vi "configuration UI.vi"() -> ()   [LabVIEW 2015, in "TDMS datalogger editor node.lvclass"]
uses:
  TDMS datalogger editor node.lvclass
  <vilib>/NI/Configuration Framework/Node/NodeRef.ctl
  <vilib>/NI/Configuration Framework/Node/NISE_CEF_Node.lvclass
  <vilib>/NI/AMC/Message Queue.ctl
  <vilib>/NI/AMC/Message.ctl
  <vilib>/NI/Tools/Keyed Array/KeyedArray.ctl
  <vilib>/NI/Configuration Framework/Node/UserEventRef.ctl
  <vilib>/NI/Configuration Framework/Controls/EventCluster.ctl
  <vilib>/NI/DCAF UI Toolkit/Controls/Move One Right.ctl
  <vilib>/NI/DCAF UI Toolkit/Controls/Move All Right.ctl
  <vilib>/NI/DCAF UI Toolkit/Controls/Move One Left.ctl
  <vilib>/NI/Configuration Framework/Node/NodeChangeEvent.ctl
  <vilib>/NI/DCAF UI Toolkit/Controls/Add.ctl
  <vilib>/NI/DCAF UI Toolkit/Controls/Remove.ctl
  <vilib>/NI/Configuration Framework/Node/RefreshUIEvent.ctl
  <vilib>/NI/Configuration Framework/Node/StopEvent.ctl
  <vilib>/NI/Configuration Framework/Node/CacheState.ctl
  <vilib>/NI/DCAF/Tag Editor Core/Table API/Available Tag Menu/channel action event.ctl
  <vilib>/NI/DCAF/Tag Editor Core/Table API/Available Tag Menu/dialog output action.ctl
  <vilib>/NI/Tag Bus Module Framework/channel/TBM channel.lvclass
  <vilib>/NI/Tag Bus/tag/tag descriptor.lvclass
  <vilib>/NI/DCAF/Tag Editor Core/Table API/Table Manager/Call Back Ref Type Def.ctl
  <vilib>/NI/DCAF/Tag Editor Core/Configuration Editor/Classes/Engine Parent/Engine Parent Editor Node.lvclass
  <vilib>/NI/DCAF/Tag Editor Core/Configuration Editor/Classes/Module editor node/module editor node.lvclass
  <vilib>/NI/DCAF UI Toolkit/Controls/Configure.ctl
  <vilib>/NI/DCAF/Tag Editor Core/Table API/Table Manager/object ref.ctl
  module/configuration/TDMS datalogger configuration.lvclass
  <vilib>/NI/DCAF/Tag Editor Core/Table API/Table Manager/references.ctl
  <vilib>/Utility/miscctls.llb/LVPositionTypeDef.ctl
  TDMS datalogger editor node.lvclass/TDMS datalogger editor node.ctl
  module/configuration/TDMS datalogger configuration.lvclass/TDMS datalogger configuration.ctl
  Write channel table.vi
  Write avail tags table.vi
  module/configuration/Read backup directory.vi
  module/configuration/Read Path.vi
  module/configuration/Read queue size.vi
  module/configuration/Read scans per write.vi
  module/configuration/Read add enable channel.vi
  module/configuration/Read channel pattern matches.vi
  module/configuration/Read log name.vi
  module/configuration/Read logrotate_options.vi
  <vilib>/NI/DCAF/Tag Editor Core/Configuration Editor/Classes/Module editor node/Read Module Configuration.vi
  <vilib>/NI/Tag Bus Module Framework/module configuration/TBM module configuration.lvclass
  <vilib>/NI/DCAF/Tag Editor Core/Table API/Listbox/Multi Column Listbox.lvclass
  <vilib>/NI/Configuration Framework/NISE_CEF_TreeControl.lvlib
  <vilib>/NI/DCAF UI Toolkit/Controls/DCAF UI Elements.lvlib
  <vilib>/NI/Tools/Keyed Array/Tools_KeyedArray.lvlib
  <vilib>/NI/AMC/AMC.lvlib
  <vilib>/NI/DCAF/Tag Editor Core/Table API/Table Manager/Table Manager.lvclass
  <vilib>/NI/DCAF/Tag Editor Core/Table API/Table Manager.lvlib
panel:
  in  "References":T1
  in  "Maximum File Size (KB)":i64=10000
  in  "user event out":refnum<user-event>
  in  "cache state":T2
  in  "stop event":T3
  in  "refresh UI":T4
  in  "node change":T5
  in  "Tab Control":T6(tab)
  in  "channels":i32(listbox)
  in  "remove":T7
  in  "avail tags":i32(listbox)=-1
  in  "add all":T8
  in  "add1":T9
  out "Logging File Path":string
  in  "file name error":bool
  in  "Log Directory":string
  in  "File Name":string
  out "Enable Tag":string
  in  "path error":bool
  in  "Use Enable Channel":bool
  in  "recalc":bool
  out "Approximate Memory Usage":dbl
  in  "Queue Size":u16=2
  in  "Scans Per Write":u16=20
  in  "Log Directory":path
  in  "Maximum Age of Files (days)":dbl=365.0
  in  "Rotate count":u32 caption="Maximum Number of Archived Files To Keep"
  in  "archive in place":bool caption="Archive Old Logs in Original Directory"
  in  "Archive Directory":string
  in  "Archive Directory":path
  in  "archive error":bool
  in  "Channel Subscription Pattern Matches":string[](array[string])
  in  "Enable Dynamic Mapping":bool
  in  "Remove Group":T10
  in  "Add Group":T11
  in  "Remove from Group":T9
  in  "Add to Group":T7
  in  "avail logged tags":i32(listbox)=-1
  in  "Groups":string(tree)="Channel1"
  in  "Add Group Name":string caption="File Name"
  in  "File Property Settings":T12
  in  "File Properties":i32(listbox)
  in  "Add File Property":T11
  in  "Remove File Property":T10
  in  "user event":T13
  in  "main queue":T14
  in  "node ref":T15
  # "kB"
  # "Note: This value ignores dynamic mapping"
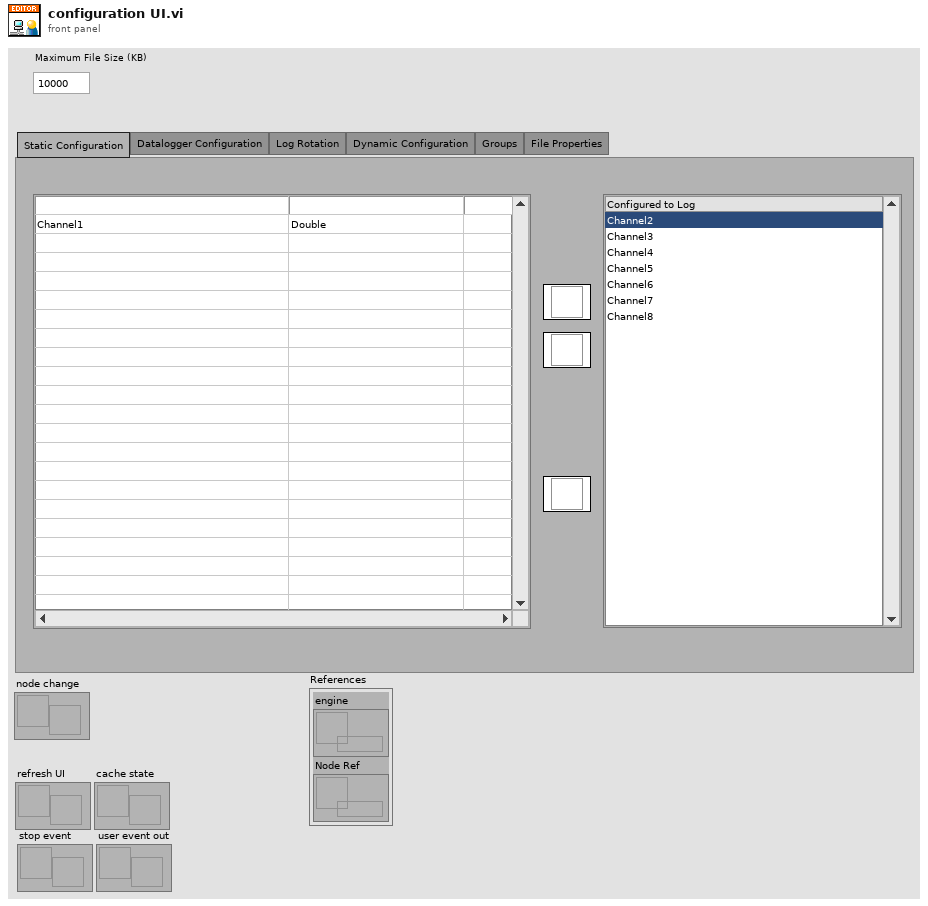
[diagram p1: front panel]
types:
  T1 = typedef "Table Manager.lvlib/Table Manager.lvclass/object ref.ctl" = cluster{"engine":refnum<data-value>, "Node Ref":refnum<data-value>}
  T2 = typedef "NISE_CEF_Node.lvclass/CacheState.ctl" = refnum<user-event>
  T3 = typedef "NISE_CEF_Node.lvclass/StopEvent.ctl" = refnum<user-event>
  T4 = typedef "NISE_CEF_Node.lvclass/RefreshUIEvent.ctl" = refnum<user-event>
  T5 = typedef "NISE_CEF_Node.lvclass/NodeChangeEvent.ctl" = refnum<user-event>
  T6 = enum32{"Static Configuration", "Datalogger Configuration", "Log Rotation", "Dynamic Configuration", "Groups", "File Properties"}
  T7 = typedef "DCAF UI Elements.lvlib/Move One Left.ctl" = bool
  T8 = typedef "DCAF UI Elements.lvlib/Move All Right.ctl" = bool
  T9 = typedef "DCAF UI Elements.lvlib/Move One Right.ctl" = bool
  T10 = typedef "DCAF UI Elements.lvlib/Remove.ctl" = bool
  T11 = typedef "DCAF UI Elements.lvlib/Add.ctl" = bool
  T12 = typedef "DCAF UI Elements.lvlib/Configure.ctl" = bool
  T13 = typedef "NISE_CEF_Node.lvclass/UserEventRef.ctl" = refnum<user-event>
  T14 = typedef "AMC.lvlib/Message Queue.ctl" = refnum<queue>
  T15 = typedef "NISE_CEF_Node.lvclass/NodeRef.ctl" = refnum<data-value>
  T16 = typedef "Table Manager.lvlib/Table Manager.lvclass/references.ctl" = cluster{"stop event":T3, "refresh UI":T4, "cache state":T2, "node change":T5, "user event out":refnum<user-event>, "main queue":T14, "user event":T13}
  T17 = typedef "LVPositionTypeDef.ctl" = cluster{"Left":i32, "Top":i32}
  T18 = typedef "TBM configuration.lvclass/Target Types.ctl" = enum16{"Windows", "Mac", "Linux", "Linux RT ARM", "VxWorks", "Pharlap", "Other", "Linux RT x64"}
  T19 = typedef "LogRotate.lvclass/options.ctl" = cluster{"max file size (bytes)":i64, "rotate count":u32, "max age (days)":dbl, "No archive dir":bool, "Archive dir":path}
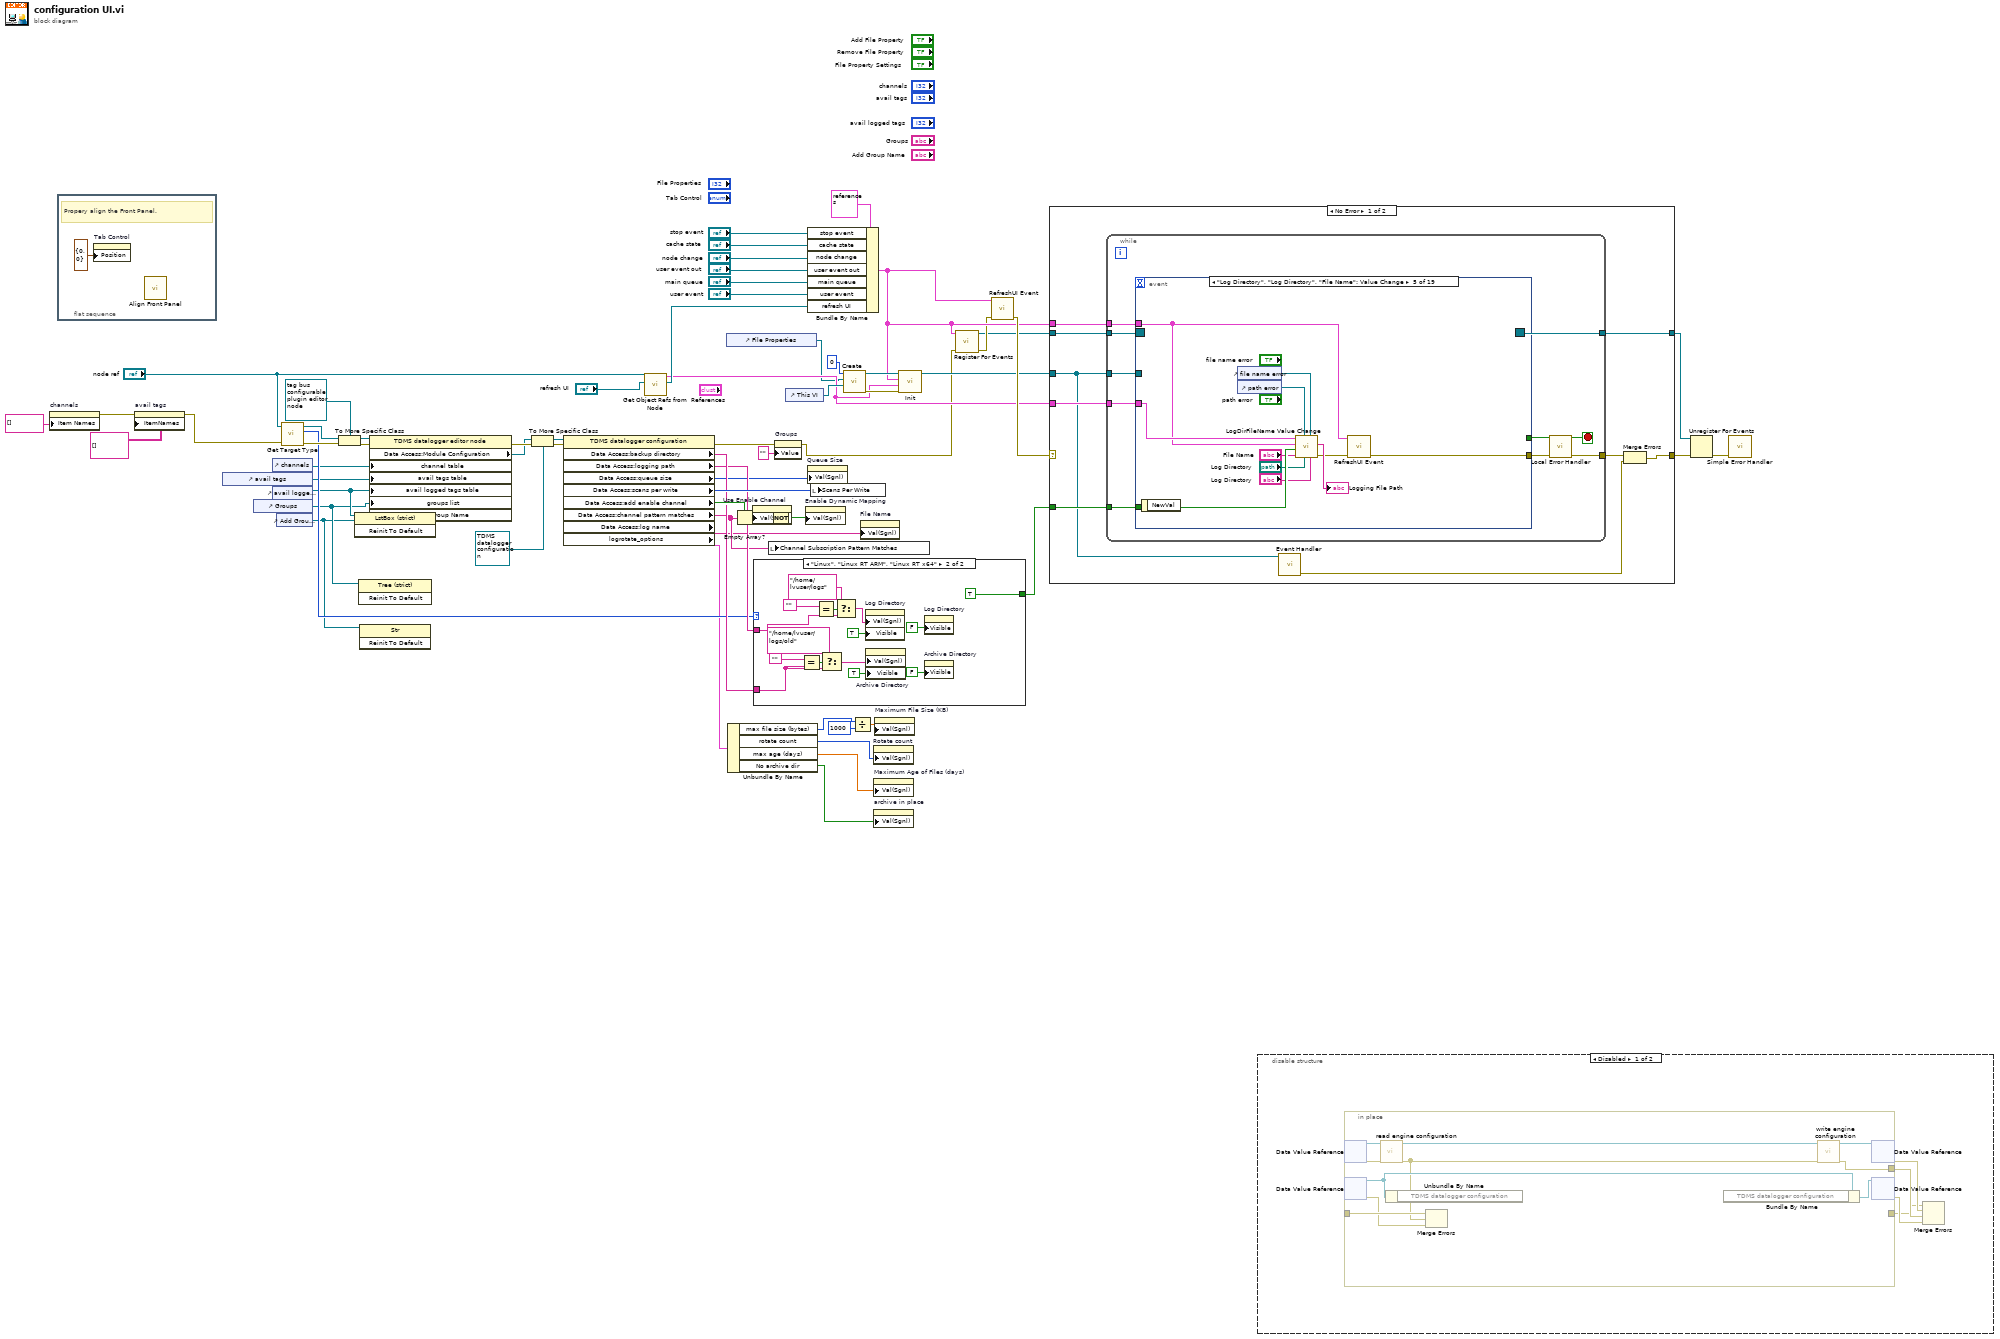
[diagram p0: block diagram]
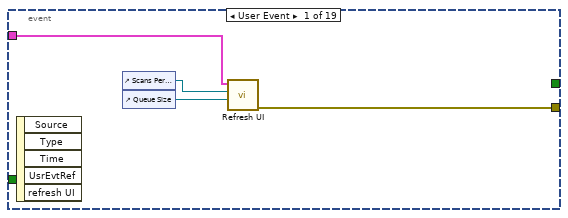
[diagram p2: hidden frame]
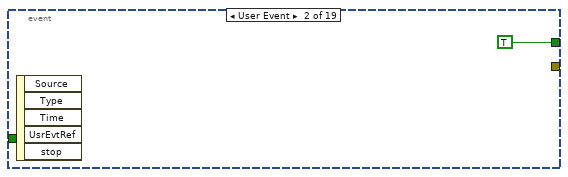
[diagram p3: hidden frame]
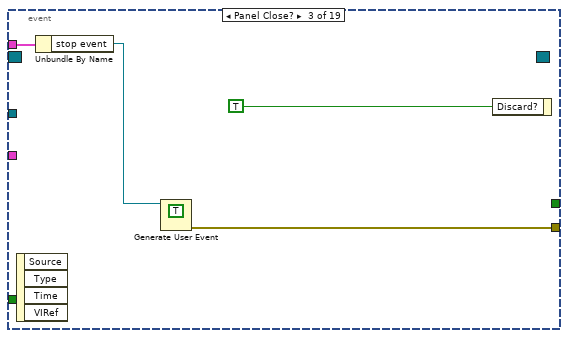
[diagram p4: hidden frame]
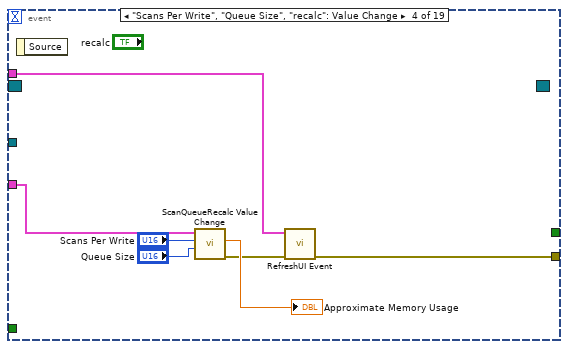
[diagram p5: hidden frame]
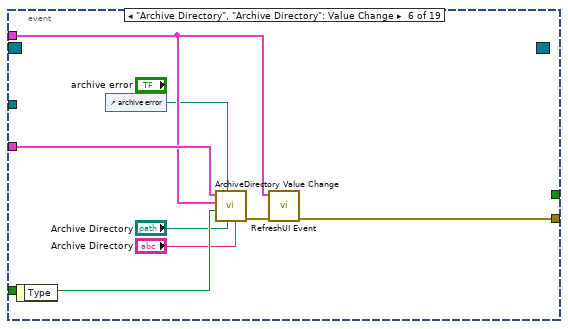
[diagram p6: hidden frame]
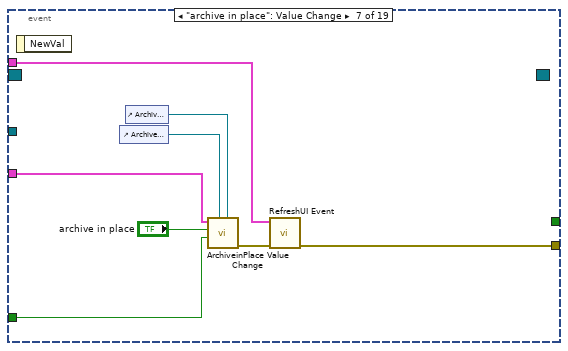
[diagram p7: hidden frame]
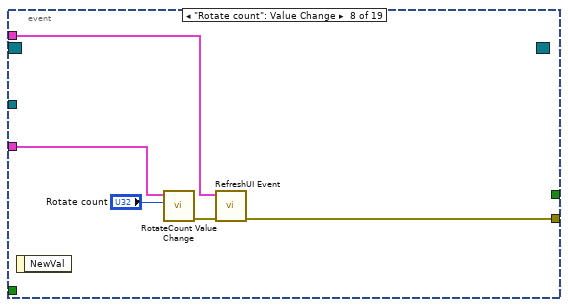
[diagram p8: hidden frame]
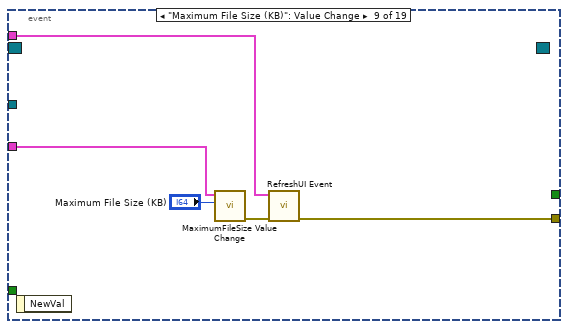
[diagram p9: hidden frame]
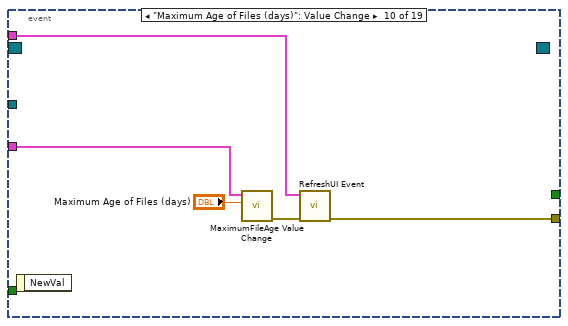
[diagram p10: hidden frame]
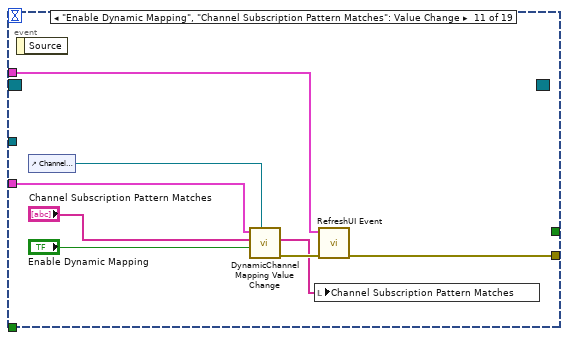
[diagram p11: hidden frame]
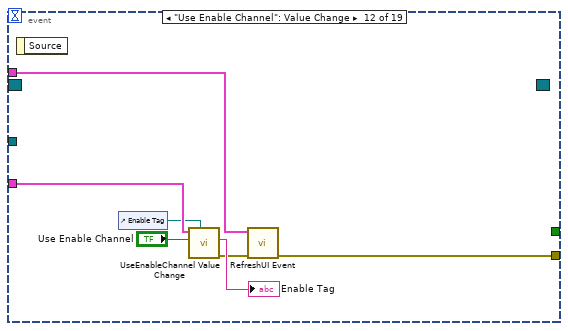
[diagram p12: hidden frame]
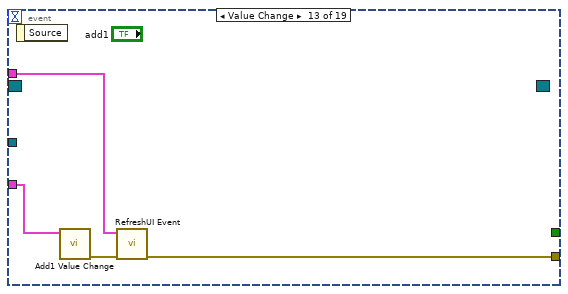
[diagram p13: hidden frame]
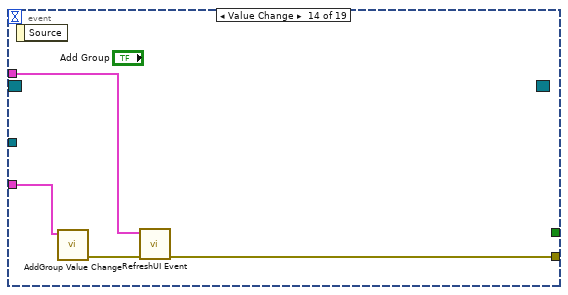
[diagram p14: hidden frame]
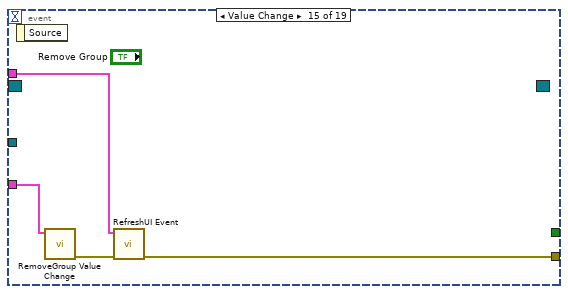
[diagram p15: hidden frame]
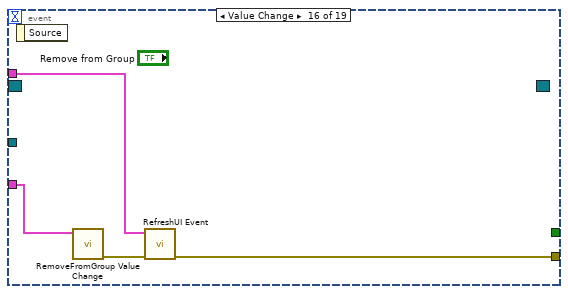
[diagram p16: hidden frame]
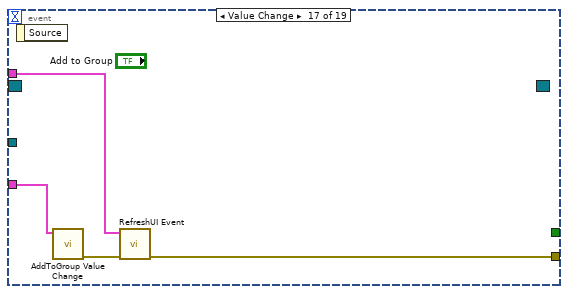
[diagram p17: hidden frame]
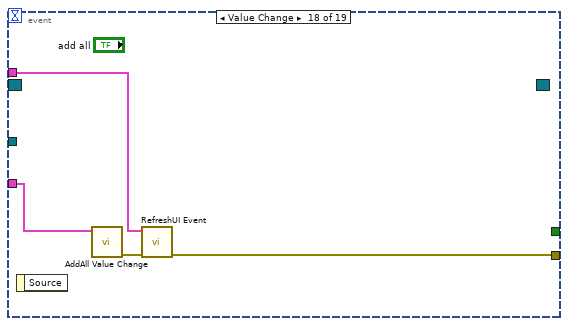
[diagram p18: hidden frame]
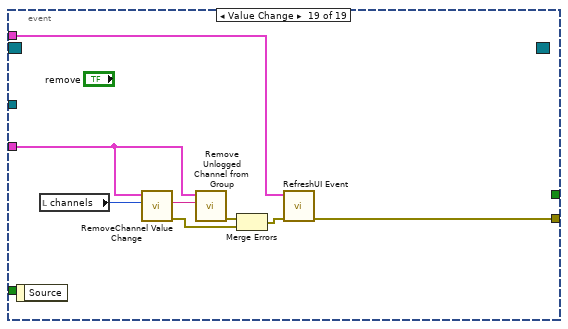
[diagram p19: hidden frame]
diagram:
  n1 = property on="channels" class="LstBox (strict)"("Item Names"=string[] []) -> (error out=w49:errorcluster)  [unwired: 2 in, 1 out]
  n2 = flat-sequence {
    frame #0 {
      # "Propery align the Front Panel."
      n3 = property on="Tab Control" class="TabCtl (strict)"("Position"=T17 {"Left"=0, "Top"=0}) -> ()  [unwired: 2 in, 2 out]
      n4 = call <vilib>:"Align Front Panel.vi"() -> ()  [unwired: 10 in, 2 out]
    }
  }
  n5 = property on="avail tags" class="MCListbox (strict)"(error in=w49, "ItemNames"=string[][] [] ("Item Names")) -> (error out=w2:errorcluster)  [unwired: 1 in, 1 out]
  n6 = control-ref of="avail tags"() -> (w36:refnum<vi>)
  n7 = control-ref of="Groups"() -> (w27:refnum<vi>)
  n8 = control-ref of="channels"() -> (w37:refnum<vi>)
  n9 = control-ref of="avail logged tags"() -> (w28:refnum<vi>)
  n10 = control-ref of="Add Group Name"() -> (w26:refnum<vi>)
  n11 = call "Get Target Type.vi"("error in (no error)"=w2, "node ref in"="node ref") -> ("error out"=w42:errorcluster, "Target Type"=w40:T18, "node ref out"=w41:T15)  [unwired: 6 in]
  n12 = To More Specific Class(target class=refnum<data-value> refnum ("data value reference"), reference=w41, error in=w42) -> (specific class reference=w45:refnum<data-value>, error out=w44:errorcluster)
  n13 = invoke class="LstBox (strict)" method="Reinit To Default"(reference=w28) -> ()  [unwired: 2 in, 3 out]
  n14 = invoke class="Tree (strict)" method="Reinit To Default"(reference=w27) -> ()  [unwired: 2 in, 3 out]
  n15 = invoke class="Str" method="Reinit To Default"(reference=w26) -> ()  [unwired: 2 in, 3 out]
  n16 = property class="TDMS datalogger editor node"(reference=w45, error in=w44, "channel table"=w37, "avail tags table"=w36, "avail logged tags table"=w28, "groups list"=w27, "Add Group Name"=w26) -> (error out=w62:errorcluster, "Data Access:Module Configuration"=w52:refnum<class "TBM module configuration.lvclass">)  [unwired: 1 out]
  n17 = To More Specific Class(target class=refnum<class "TDMS datalogger configuration.lvclass"> refnum ("TDMS datalogger configuration"), reference=w52, error in=w62) -> (specific class reference=w50:refnum<class "TDMS datalogger configuration.lvclass">, error out=w53:errorcluster)
  n18 = property class="TDMS datalogger configuration"(reference=w50, error in=w53) -> (error out=w24:errorcluster, "Data Access:backup directory"=w59:string, "Data Access:logging path"=w58:string, "Data Access:queue size"=w57:u16, "Data Access:scans per write"=w61:u16, "Data Access:add enable channel"=w60:bool, "Data Access:channel pattern matches"=w56:string[], "Data Access:log name"=w39:string, "logrotate_options"=w35:T19)  [unwired: 1 out]
  n19 = call "Get Object Refs from Node.vi"("Refresh UI"="refresh UI", "node ref"="node ref") -> ("Refresh UI out"=w9:T4, "References"=w8:T1)  [unwired: 7 in, 1 out]
  n20 = control-ref of="File Properties"() -> (w7:refnum<vi>)
  n21 = Unbundle By Name(w35) -> ("max file size (bytes)"=w31:i64, "rotate count"=w33:u32, "max age (days)"=w34:dbl, "No archive dir"=w32:bool)
  n22 = Empty Array?(array=w56) -> (empty?=w54:bool)
  n23 = property on="Use Enable Channel" class="Bool (strict)"("Val(Sgnl)"=w60) -> ()  [unwired: 2 in, 2 out]
  n24 = case shown="\"Linux\", \"Linux RT ARM\", \"Linux RT x64\"" w40 {
    tunnel: w59 -> [w67 w86]
    tunnel: w58 -> [w76 w93]
    tunnel: [FALSE TRUE] -> w38
    frame Default {
      w83 = FALSE ("Visible")
      n25 = call <vilib>:"Dflt Data Dir.vi"() -> ("App:Default Data Directory"=w79:path)
      n26 = call <vilib>:"Dflt Data Dir.vi"() -> ("App:Default Data Directory"=w70:path)
      n27 = Build Path(base path=w79, name or relative path="logs") -> (appended path=w81:path)
      n28 = Build Path(base path=w70, name or relative path="logs\\old") -> (appended path=w68:path)
      n29 = String To Path(string=w76) -> (path=w75:path)
      n30 = Equal?(x="", y=w76) -> (x = y?=w77:bool)
      n31 = String To Path(string=w67) -> (path=w73:path)
      n32 = Equal?(x="", y=w67) -> (x = y?=w72:bool)
      n33 = Select(t=w81, s=w77, f=w75) -> (s? t:f=w74:path)
      n34 = Select(t=w68, s=w72, f=w73) -> (s? t:f=w66:path)
      n35 = property on="Archive Directory" class="Path"("Val(Sgnl)"=w66, "Visible"=TRUE) -> ()  [unwired: 2 in, 2 out]
      n36 = property on="Log Directory" class="Path"("Val(Sgnl)"=w74, "Visible"=TRUE) -> ()  [unwired: 2 in, 2 out]
      n37 = property on="Archive Directory" class="Str"("Visible"=w83) -> ()  [unwired: 2 in, 2 out]
      n38 = property on="Log Directory" class="Str"("Visible"=w83) -> ()  [unwired: 2 in, 2 out]
    }
    frame "Linux", "Linux RT ARM", "Linux RT x64" {
      n39 = Equal?(x="", y=w86) -> (x = y?=w89:bool)
      n40 = Equal?(x="", y=w93) -> (x = y?=w94:bool)
      n41 = Select(t="/home/lvuser/logs/old", s=w89, f=w86) -> (s? t:f=w87:string)
      n42 = Select(t="/home/lvuser/logs", s=w94, f=w93) -> (s? t:f=w92:string)
      n43 = property on="Log Directory" class="Str"("Val(Sgnl)"=w92, "Visible"=TRUE) -> ()  [unwired: 2 in, 2 out]
      n44 = property on="Archive Directory" class="Str"("Val(Sgnl)"=w87, "Visible"=TRUE) -> ()  [unwired: 2 in, 2 out]
      n45 = property on="Log Directory" class="Path"("Visible"=FALSE) -> ()  [unwired: 2 in, 2 out]
      n46 = property on="Archive Directory" class="Path"("Visible"=FALSE) -> ()  [unwired: 2 in, 2 out]
    }
  }
  n47 = local write "Channel Subscription Pattern Matches"(w56) -> ()
  n48 = Not(x=w54) -> (.not. x?=w55:bool)
  n49 = property on="Groups" class="Tree (strict)"(error in=w24, "Value"="" ("Groups")) -> (error out=w4:errorcluster)  [unwired: 1 in, 1 out]
  n50 = control-ref of="This VI"() -> (w14:refnum<vi>)
  n51 = property on="Enable Dynamic Mapping" class="Bool (strict)"("Val(Sgnl)"=w55) -> ()  [unwired: 2 in, 2 out]
  n52 = Bundle By Name(cluster=T16 {"stop event"=refnum, "refresh UI"=refnum, "cache state"=refnum, "node change"=refnum, "user event out"=refnum, "main queue"=refnum, "user event"=refnum} ("References"), "stop event"="stop event", "cache state"="cache state", "node change"="node change", "user event out"="user event out", "main queue"="main queue", "user event"="user event", "refresh UI"=w9) -> (w6:T16)
  n53 = property on="Queue Size" class="DigNum (strict)"("Val(Sgnl)"=w57) -> ()  [unwired: 2 in, 2 out]
  n54 = local write "Scans Per Write"(w61) -> ()
  n55 = call <vilib>:"Create.vi"("Top VI"=w14, "Listbox"=w7, "Index"=0) -> ("error out"=w12:errorcluster, "reference out"=w13:refnum<class "Multi Column Listbox.lvclass">)  [unwired: 7 in]
  n56 = Divide(x=w31, y=i64 1000) -> (x/y=w30:dbl)
  n57 = property on="File Name" class="Str"("Val(Sgnl)"=w39) -> ()  [unwired: 2 in, 2 out]
  n58 = property on="Rotate count" class="DigNum (strict)"("Val(Sgnl)"=w33) -> ()  [unwired: 2 in, 2 out]
  n59 = property on="Maximum Age of Files (days)" class="DigNum (strict)"("Val(Sgnl)"=w34) -> ()  [unwired: 2 in, 2 out]
  n60 = property on="archive in place" class="Bool (strict)"("Val(Sgnl)"=w32) -> ()  [unwired: 2 in, 2 out]
  n61 = property on="Maximum File Size (KB)" class="DigNum (strict)"("Val(Sgnl)"=w30) -> ()  [unwired: 2 in, 2 out]
  n62 = call-dynamic "Init.vi"("error in (no error)"=w12, "Node object refs"=w8, "Event References"=w6, "Multi Column Listbox in"=w13) -> ("Multi Column Listbox out"=w10:refnum<class "Multi Column Listbox.lvclass">)  [unwired: 5 in, 2 out]
  n63 = call "Register For Events.vi"("error in"=w4, "References"=w6) -> ("error out"=w5:errorcluster, "Event Registration Refnum"=w3:refnum<event-registration>)  [unwired: 8 in]
  n64 = call "RefreshUI Event.vi"("error in (no error)"=w5, "References in"=w6) -> ("error out"=w11:errorcluster)  [unwired: 8 in, 1 out]
  n65 = case shown="No Error" w11 {
    selector: w11 -> [_ w227]
    tunnel: w3 -> [w109 w226]
    tunnel: [w108 w226] -> w64
    tunnel: [w102 w227] -> w46
    tunnel: w38 -> [w106 _]
    tunnel: w8 -> [w105 _]
    tunnel: w10 -> [w104 _]
    tunnel: w6 -> [w103 _]
    frame No Error {
      n66 = while {
        tunnel: w109 -> [w119]
        tunnel: [w118] -> w108
        tunnel: [w112] -> w107
        tunnel: w106 -> [w117]
        tunnel: w105 -> [w116]
        tunnel: w104 -> [w115]
        tunnel: w103 -> [w114]
        stop <- w110 stop-if-true
        n67 = event shown="[4] \"Log Directory\", \"Log Directory\", \"File Name\": Value Change" {
          selector: w119 -> [_ _ _ _ _ _ _ _ _ _ _ _ _ _ _ _ _ _ _]
          dyn-events: [_ _ _ _ _ _ _ _ _ _ _ _ _ _ _ _ _ _ _] -> w118
          timeout: _ -> [_ _ _ _ _ _ _ _ _ _ _ _ _ _ _ _ _ _ _]
          tunnel: [_ TRUE _ _ _ _ _ _ _ _ _ _ _ _ _ _ _ _ _] -> w111
          tunnel: [w122 _ w128 w131 w137 w155 w156 w165 w170 w174 w184 w187 w194 w199 w203 w206 w210 w214 w222] -> w113
          tunnel: w117 -> [_ _ _ _ w145 w151 w162 _ _ _ _ _ _ _ _ _ _ _ _]
          tunnel: w116 -> [w123 _ _ w135 w147 w154 w161 w167 w172 w176 w182 w192 w196 w198 w204 w208 w212 w216 w221]
          tunnel: w115 -> [_ _ _ _ _ _ _ _ _ _ _ _ _ _ _ _ _ _ _]
          tunnel: w114 -> [_ _ w127 w136 w146 w153 w163 w168 w169 w178 w186 w193 w197 w201 w205 w209 w213 w217 w225]
          event User Event {
            n68 = event-data() -> ()  [unwired: 1 in, 5 out]
            n69 = control-ref of="Scans Per Write"() -> (w121:refnum<vi>)
            n70 = control-ref of="Queue Size"() -> (w120:refnum<vi>)
            n71 = call "Refresh UI.vi"("Queue Size ref"=w120, "Scans Per Write ref"=w121, "References"=w123) -> ("error out"=w122:errorcluster)  [unwired: 8 in]
          }
          event User Event {
            n72 = event-data() -> ()  [unwired: 1 in, 5 out]
          }
          event Panel Close? {
            n73 = event-data() -> ()  [unwired: 1 in, 4 out]
            n74 = Unbundle By Name(w127) -> ("stop event"=w126:T3)
            n75 = Generate User Event(user event=w126, event data cluster=TRUE ("event data")) -> (error out=w128:errorcluster)  [unwired: 2 in, 1 out]
            n76 = event-data("Discard?"=TRUE) -> ()  [unwired: 1 in, 1 out]
          }
          event "Scans Per Write", "Queue Size", "recalc": Value Change {
            n77 = event-data() -> ()  [unwired: 1 in, 1 out]
            n78 = call "ScanQueueRecalc Value Change.vi"("Queue Size"="Queue Size", "Scans Per Write"="Scans Per Write", "References"=w135) -> ("error out"=w130:errorcluster, "Approximate Memory Usage"=→"Approximate Memory Usage":dbl)  [unwired: 7 in]
            n79 = call "RefreshUI Event.vi"("error in (no error)"=w130, "References in"=w136) -> ("error out"=w131:errorcluster)  [unwired: 8 in, 1 out]
          }
          event "Log Directory", "Log Directory", "File Name": Value Change {
            n80 = event-data() -> ()  [unwired: 1 in, 1 out]
            n81 = control-ref of="file name error"() -> (w139:refnum<vi>)
            n82 = control-ref of="path error"() -> (w140:refnum<vi>)
            n83 = call "LogDirFileName Value Change.vi"("Linux Log Directory"="Log Directory", "file name error ref"=w139, "Windows Log Directory"="Log Directory", "path error ref"=w140, "File Name"="File Name", "Linux Paths?"=w145, "Event References"=w146, "References"=w147) -> ("error out"=w138:errorcluster, "Logging File Path"=→"Logging File Path":string)  [unwired: 2 in]
            n84 = call "RefreshUI Event.vi"("error in (no error)"=w138, "References in"=w146) -> ("error out"=w137:errorcluster)  [unwired: 8 in, 1 out]
          }
          event "Archive Directory", "Archive Directory": Value Change {
            n85 = event-data() -> ()  [unwired: 1 in, 1 out]
            n86 = control-ref of="archive error"() -> (w152:refnum<vi>)
            n87 = call "ArchiveDirectory Value Change.vi"("Linux Archive Directory"="Archive Directory", "Windows Archive Directory"="Archive Directory", "Archive Error ref"=w152, "Linux Paths?"=w151, "Event References"=w153, "References"=w154) -> ("error out"=w148:errorcluster)  [unwired: 5 in]
            n88 = call "RefreshUI Event.vi"("error in (no error)"=w148, "References in"=w153) -> ("error out"=w155:errorcluster)  [unwired: 8 in, 1 out]
          }
          event "archive in place": Value Change {
            n89 = event-data() -> ()  [unwired: 1 in, 1 out]
            n90 = control-ref of="Archive Directory"() -> (w159:refnum<vi>)
            n91 = control-ref of="Archive Directory"() -> (w160:refnum<vi>)
            n92 = call "ArchiveinPlace Value Change.vi"("Windows archive path ref"=w160, "Linux archive path reference"=w159, "Linux?"=w162, "archive in place"="archive in place", "References"=w161) -> ("error out"=w157:errorcluster)  [unwired: 6 in]
            n93 = call "RefreshUI Event.vi"("error in (no error)"=w157, "References in"=w163) -> ("error out"=w156:errorcluster)  [unwired: 8 in, 1 out]
          }
          event "Rotate count": Value Change {
            n94 = event-data() -> ()  [unwired: 1 in, 1 out]
            n95 = call "RotateCount Value Change.vi"("Rotate count"="Rotate count", "References"=w167) -> ("error out"=w166:errorcluster)  [unwired: 9 in]
            n96 = call "RefreshUI Event.vi"("error in (no error)"=w166, "References in"=w168) -> ("error out"=w165:errorcluster)  [unwired: 8 in, 1 out]
          }
          event "Maximum File Size (KB)": Value Change {
            n97 = event-data() -> ()  [unwired: 1 in, 1 out]
            n98 = call "MaximumFileSize Value Change.vi"("Maximum File Size (KB)"="Maximum File Size (KB)", "References"=w172) -> ("error out"=w171:errorcluster)  [unwired: 9 in]
            n99 = call "RefreshUI Event.vi"("error in (no error)"=w171, "References in"=w169) -> ("error out"=w170:errorcluster)  [unwired: 8 in, 1 out]
          }
          event "Maximum Age of Files (days)": Value Change {
            n100 = event-data() -> ()  [unwired: 1 in, 1 out]
            n101 = call "MaximumFileAge Value Change.vi"("Maximum Age of Files (days)"="Maximum Age of Files (days)", "References"=w176) -> ("error out"=w175:errorcluster)  [unwired: 9 in]
            n102 = call "RefreshUI Event.vi"("error in (no error)"=w175, "References in"=w178) -> ("error out"=w174:errorcluster)  [unwired: 8 in, 1 out]
          }
          event "Enable Dynamic Mapping", "Channel Subscription Pattern Matches": Value Change {
            n103 = event-data() -> ()  [unwired: 1 in, 1 out]
            n104 = control-ref of="Channel Subscription Pattern Matches"() -> (w179:refnum<vi>)
            n105 = call "DynamicChannelMapping Value Change.vi"("Channel Pattern Matches ref"=w179, "Enable Dynamic Mapping"="Enable Dynamic Mapping", "Channel Subscription Pattern Matches"="Channel Subscription Pattern Matches", "References"=w182) -> ("error out"=w185:errorcluster, "Patter Matches out"=w180:string[])  [unwired: 6 in]
            n106 = local write "Channel Subscription Pattern Matches"(w180) -> ()
            n107 = call "RefreshUI Event.vi"("error in (no error)"=w185, "References in"=w186) -> ("error out"=w184:errorcluster)  [unwired: 8 in, 1 out]
          }
          event "Use Enable Channel": Value Change {
            n108 = event-data() -> ()  [unwired: 1 in, 1 out]
            n109 = control-ref of="Enable Tag"() -> (w190:refnum<vi>)
            n110 = call "UseEnableChannel Value Change.vi"("Enable Tag ref"=w190, "Use Enable Channel"="Use Enable Channel", "References"=w192) -> ("error out"=w188:errorcluster, "Enable Tag"=→"Enable Tag":string)  [unwired: 7 in]
            n111 = call "RefreshUI Event.vi"("error in (no error)"=w188, "References in"=w193) -> ("error out"=w187:errorcluster)  [unwired: 8 in, 1 out]
          }
          event Value Change {
            n112 = event-data() -> ()  [unwired: 1 in, 1 out]
            n113 = call "Add1 Value Change.vi"("References"=w196) -> ("error out"=w195:errorcluster)  [unwired: 10 in]
            n114 = call "RefreshUI Event.vi"("error in (no error)"=w195, "References in"=w197) -> ("error out"=w194:errorcluster)  [unwired: 8 in, 1 out]
          }
          event Value Change {
            n115 = event-data() -> ()  [unwired: 1 in, 1 out]
            n116 = call "AddGroup Value Change.vi"("References"=w198) -> ("error out"=w200:errorcluster)  [unwired: 10 in]
            n117 = call "RefreshUI Event.vi"("error in (no error)"=w200, "References in"=w201) -> ("error out"=w199:errorcluster)  [unwired: 8 in, 1 out]
          }
          event Value Change {
            n118 = event-data() -> ()  [unwired: 1 in, 1 out]
            n119 = call "RemoveGroup Value Change.vi"("References"=w204) -> ("error out"=w202:errorcluster)  [unwired: 10 in]
            n120 = call "RefreshUI Event.vi"("error in (no error)"=w202, "References in"=w205) -> ("error out"=w203:errorcluster)  [unwired: 8 in, 1 out]
          }
          event Value Change {
            n121 = event-data() -> ()  [unwired: 1 in, 1 out]
            n122 = call "RemoveFromGroup Value Change.vi"("References"=w208) -> ("error out"=w207:errorcluster)  [unwired: 10 in]
            n123 = call "RefreshUI Event.vi"("error in (no error)"=w207, "References in"=w209) -> ("error out"=w206:errorcluster)  [unwired: 8 in, 1 out]
          }
          event Value Change {
            n124 = event-data() -> ()  [unwired: 1 in, 1 out]
            n125 = call "AddToGroup Value Change.vi"("References"=w212) -> ("error out"=w211:errorcluster)  [unwired: 10 in]
            n126 = call "RefreshUI Event.vi"("error in (no error)"=w211, "References in"=w213) -> ("error out"=w210:errorcluster)  [unwired: 8 in, 1 out]
          }
          event Value Change {
            n127 = event-data() -> ()  [unwired: 1 in, 1 out]
            n128 = call "AddAll Value Change.vi"("References"=w216) -> ("error out"=w215:errorcluster)  [unwired: 10 in]
            n129 = call "RefreshUI Event.vi"("error in (no error)"=w215, "References in"=w217) -> ("error out"=w214:errorcluster)  [unwired: 8 in, 1 out]
          }
          event Value Change {
            n130 = event-data() -> ()  [unwired: 1 in, 1 out]
            n131 = local read "channels"() -> (w224:i32)
            n132 = call "RemoveChannel Value Change.vi"("channel"=w224, "References"=w221) -> ("error out"=w223:errorcluster, "Removed Channel Name"=w220:string)  [unwired: 8 in]
            n133 = call "Remove Unlogged Channel from Group.vi"("Item Name"=w220, "References"=w221) -> ("error out"=w218:errorcluster)  [unwired: 9 in]
            n134 = Merge Errors(w218, w223) -> (w219:errorcluster)
            n135 = call "RefreshUI Event.vi"("error in (no error)"=w219, "References in"=w225) -> ("error out"=w222:errorcluster)  [unwired: 8 in, 1 out]
          }
        }
        n136 = call "Local Error Handler.vi"("error in"=w113, "Stop in"=w111) -> ("error out"=w112:errorcluster, "Stop out"=w110:bool)  [unwired: 8 in]
      }
      n137 = call-dynamic "Event Handler.vi"("Listbox in"=w104) -> ("error out"=w101:errorcluster)  [unwired: 9 in, 1 out]
      n138 = Merge Errors(w107, w101) -> (w102:errorcluster)
    }
    frame Error {
    }
  }
  n139 = disable-structure shown="Disabled" {
    frame Disabled {
      n140 = in-place {
        in-place-border: _ -> [w241]
        in-place-border: [_] -> w228
        in-place-border: [w234] -> w229
        n141 = in-place-dvr #1() -> (w236:refnum<class "Engine Parent Editor Node.lvclass">, w237:errorcluster)  [unwired: 1 in]
        n142 = in-place-dvr #2() -> (w233:refnum<class "TDMS datalogger editor node.lvclass">, w239:errorcluster)  [unwired: 1 in]
        n143 = call <vilib>:"read engine configuration.vi"("error in"=w237, "Engine Parent Editor Node in"=w236) -> ("error out"=w232:errorcluster, "Engine Parent Editor Node out"=w235:refnum<class "Engine Parent Editor Node.lvclass">)  [unwired: 7 in, 1 out]
        n144 = Unbundle By Name(w233) -> ()  [unwired: 1 out]
        n145 = Merge Errors(w241, w232, w239) -> ()  [unwired: 1 out]
        n146 = Bundle By Name(cluster=w233) -> (w240:refnum<class "TDMS datalogger editor node.lvclass">)  [unwired: 1 in]
        n147 = call <vilib>:"write engine configuration.vi"("error in"=w232, "Engine Parent Editor Node in"=w235) -> ("error out"=w234:errorcluster, "Engine Parent Editor Node out"=w238:refnum<class "Engine Parent Editor Node.lvclass">)  [unwired: 8 in]
        n148 = in-place-dvr #1(w238) -> (w230:errorcluster)  [unwired: 1 out]
        n149 = in-place-dvr #2(w240) -> (w231:errorcluster)  [unwired: 1 out]
      }
      n150 = Merge Errors(w228, w230, w229, w231) -> ()  [unwired: 1 out]
    }
    frame Enabled {
    }
  }
  n151 = Unregister For Events(event registration refnum=w64, error in=w46) -> (error out=w63:errorcluster)
  n152 = call <vilib>:"Simple Error Handler.vi"("error in (no error)"=w63) -> ()  [unwired: 4 in, 5 out]
